vi "Write Binary.vi"(8 "error in (no error)":errorcluster, 9 "timeout ms (5000)":i32=5000, 10 "Binary Data":u8[](array[numeric]), 11 "WebSocket in":refnum<class "WebSocket.lvclass">) -> (0 "error out":errorcluster, 3 "WebSocket out":refnum<class "WebSocket.lvclass">)   [LabVIEW 2021, in "WebSockets.lvlib" / "WebSocket.lvclass"]
doc: "Writes a binary frame to the WebSocket connection endpoint.\nWebSockets 2.0.1.40\nSam Sharp - MediaMongrels Ltd\nCopyright (c) 2019, MediaMongrels Ltd"
uses:
  WebSocket.lvclass
  Opcodes.ctl
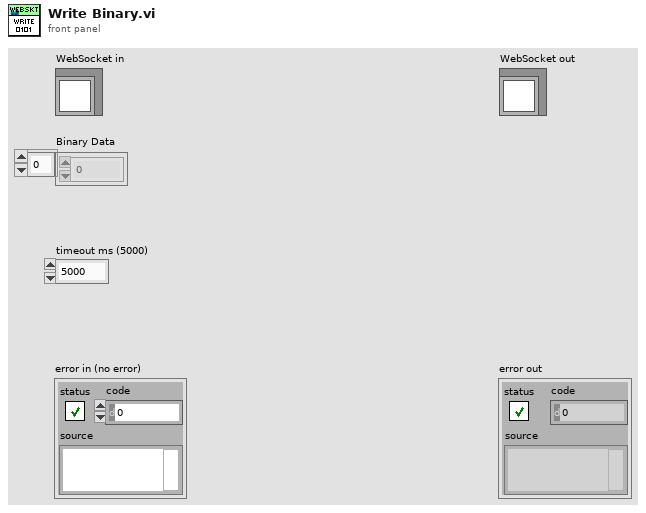
[diagram p1: front panel]
types:
  T1 = typedef "WebSockets.lvlib/WebSocket.lvclass/Opcodes.ctl" = u8
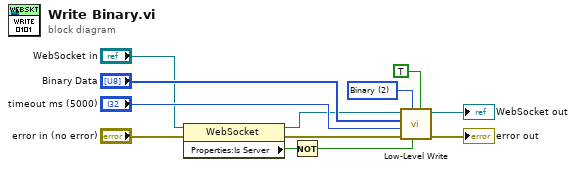
[diagram p0: block diagram]
diagram:
  w7 = T1 2 items=["Cont. Frame"=0, "Text"=1, "Binary"=2, "Close Frame"=8, "Ping"=9, "Pong"=10] ("Opcode (Text)")
  n1 = property class="WebSocket"(reference="WebSocket in", error in="error in (no error)") -> (reference out=w1:refnum<class "WebSocket.lvclass">, error out=w2:errorcluster, "Properties:Is Server"=w6:bool)
  n2 = Not(x=w6) -> (.not. x?=w3:bool)
  n3 = call "Low-Level Write.vi"("Finished? (True)"=TRUE, "Mask payload?"=w3, "Opcode (Text)"=w7, "error in (no error)"=w2, "timeout ms (5000)"="timeout ms (5000)", "Data"="Binary Data", "WebSockets in"=w1) -> ("error out"=→"error out":errorcluster, "WebSockets out"=→"WebSocket out":refnum<class "WebSocket.lvclass">)  [unwired: 3 in]
